vi "GetImage.vi"(8 "error in (no error)":errorcluster, 11 "GEECS_Image in":refnum<class "GEECS_Image.lvclass">) -> (0 "error out":errorcluster, 2 "Image Out":T1, 3 "GEECS_Image out":refnum<class "GEECS_Image.lvclass">)   [LabVIEW 2020, in "GEECS_Image.lvclass"]
uses:
  GEECS_Image.lvclass
  IMAQ Image.ctl
  GEECS_Image.lvclass/GEECS_Image.ctl
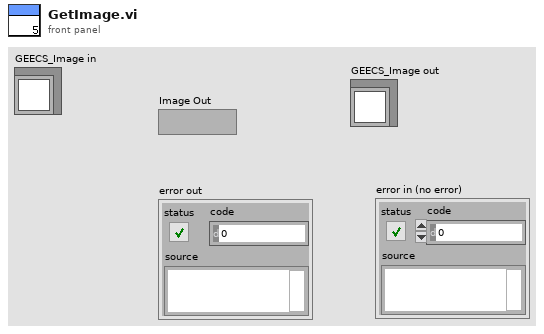
[diagram p1: front panel]
types:
  T1 = typedef "IMAQ Image.ctl" = refnum<image>
  T2 = typedef "SubscriberCluster_TypDEf.ctl" = cluster{"tcp data event":T3, "Event Registration Refnum":refnum<event-registration>, "data queue":refnum<queue>, "Devices":string[], "Alias":string[], "Variable header":string[], "Devices ALL":string[]}
  T3 = typedef "tcp_new_data_event.ctl" = refnum<user-event>
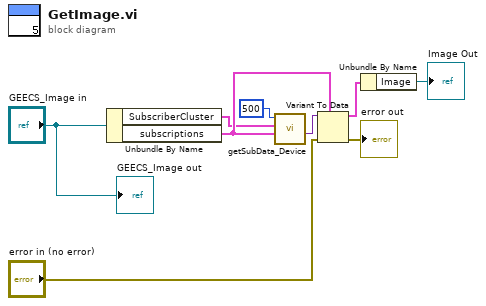
[diagram p0: block diagram]
diagram:
  n1 = Unbundle By Name("GEECS_Image in") -> ("SubscriberCluster"=w5:T2, "subscriptions"=w6:cluster{"Image":T1})
  n2 = call "getSubData_Device.vi"("variant in"=w6, "SubscriberCluster"=w5, "timeout"=500) -> ("variant out"=w4:variant)  [unwired: 6 in, 2 out]
  n3 = Variant To Data(error in="error in (no error)", type=w6, Variant=w4) -> (data=w8:cluster{"Image":T1}, error out=→"error out":errorcluster)
  n4 = Unbundle By Name(w8) -> ("Image"=→"Image Out":T1)
  "GEECS_Image out" <- "GEECS_Image in"
